vi "Day 16-Hex to Bits Map.vi"() -> (3 "Map":map{string, string}(c390))   [LabVIEW 2021]
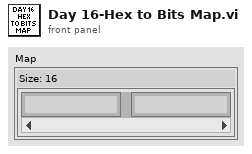
[diagram p1: front panel]
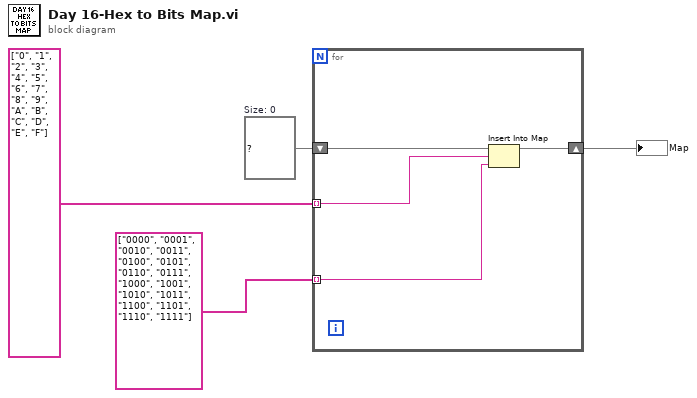
[diagram p0: block diagram]
diagram:
  w3 = map{string, string} {}  # Size: 0
  n1 = for {
    tunnel: string[] ["0", "1", "2", "3", "4", "5", "6", "7", "8", "9", "A", "B", "C", "D", "E", "F"] -> [w8] mode=indexing
    tunnel: string[] ["0000", "0001", "0010", "0011", "0100", "0101", "0110", "0111", "1000", "1001", "1010", "1011", "1100", "1101", "1110", "1111"] -> [w7] mode=indexing
    shift-right: [w6] -> w4
    shift-left: w3 -> [w5]
    n2 = Insert Into Map(map in=w5, key=w8, value=w7) -> (map out=w6:map{string, string})  [unwired: 2 out]
  }
  "Map" <- w4
